vi "3.-Bundle y Cluster.vi"() -> ()   [LabVIEW 2020]
panel:
  out "Cluster 4":T1 {"Slide" scale=0.0..10.0}
  in  "stop":bool
  out "Cluster 3":T1 {"Slide" scale=0.0..10.0}
  in  "Cluster 2":T1 {"Slide" scale=0.0..10.0}
  in  "Cluster":T1 {"Slide" scale=0.0..10.0}
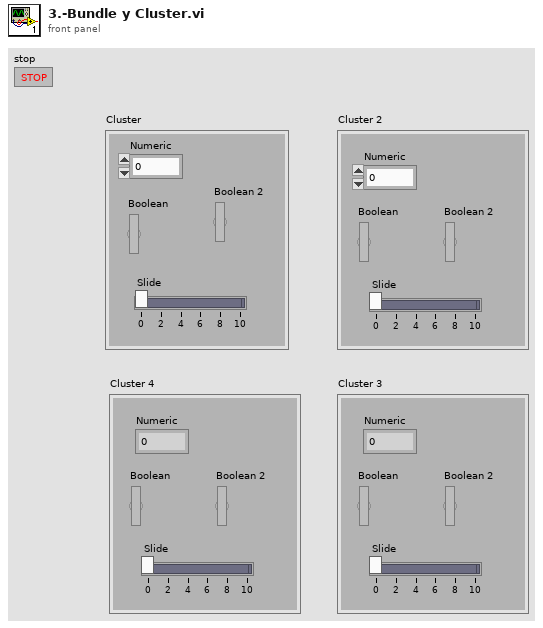
[diagram p1: front panel]
types:
  T1 = cluster{"Numeric":dbl, "Boolean":bool, "Boolean 2":bool, "Slide":dbl}
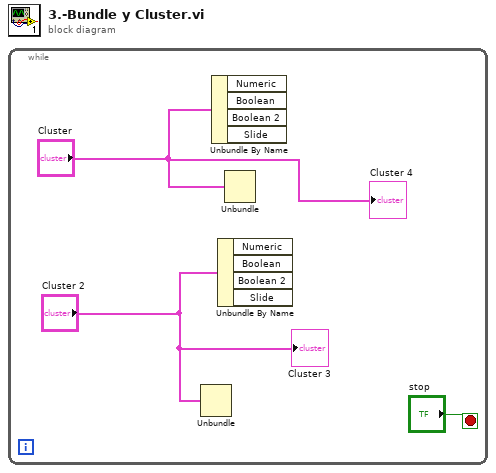
[diagram p0: block diagram]
diagram:
  n1 = while {
    stop <- "stop" stop-if-true
    n2 = Unbundle("Cluster 2") -> ()  [unwired: 4 out]
    n3 = Unbundle By Name("Cluster") -> ()  [unwired: 4 out]
    n4 = Unbundle By Name("Cluster 2") -> ()  [unwired: 4 out]
    n5 = Unbundle("Cluster") -> ()  [unwired: 4 out]
    "Cluster 3" <- "Cluster 2"
    "Cluster 4" <- "Cluster"
  }
